vi "Array to temp.vi"(10 "Array":u8[](array[numeric])) -> (2 "Temperature":sgl)   [LabVIEW 2014]
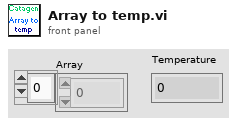
[diagram p1: front panel]
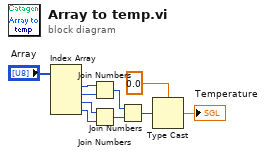
[diagram p0: block diagram]
diagram:
  n1 = Index Array(array="Array") -> (element #1=w9:u8, element #2=w8:u8, element #3=w7:u8, element #4=w6:u8)  [unwired: 4 in]
  n2 = Join Numbers(hi=w9, lo=w8) -> ((hi.lo)=w4:u16)
  n3 = Join Numbers(hi=w7, lo=w6) -> ((hi.lo)=w5:u16)
  n4 = Join Numbers(hi=w4, lo=w5) -> ((hi.lo)=w3:u32)
  n5 = Type Cast(type=sgl 0.0, x=w3) -> (*(type *) &x=→"Temperature":sgl)
